vi "FABR-Init Hardware.vi"(0 "Stimulus":T1={"Ear"=enum."Left", "Start (kHz)"=0.0, "Stop (kHz)"=16.0, "Step (oct)"=5.0, "Start (dB)"=20, "Stop (dB)"=80, "Step (dB)"=5, "Rep rate (/sec)"=30.0, "Alternate Polarity"=FALSE, "Skip (oct)"=0.0} {"Start (kHz)" step=5.0; "Start (dB)" step=5}, 9 "Hidden":T3={"AI Samp Rate Hz"=25000.0, "AO Samp Rate Hz"=100000.0, "Duration (ms)"=5.0, "Ramp (ms)"=0.5, "Frame size (s)"=0.0}, 11 "error in (no error)":errorcluster) -> (4 "Stimulus thru":T1={"Ear"=enum."Left", "Start (kHz)"=0.0, "Stop (kHz)"=16.0, "Step (oct)"=5.0, "Start (dB)"=20, "Stop (dB)"=80, "Step (dB)"=5, "Rep rate (/sec)"=30.0, "Alternate Polarity"=FALSE, "Skip (oct)"=0.0} {"Start (kHz)" step=5.0; "Start (dB)" step=5}, 6 "Runtime":T2, 8 "Coerced rep rate":dbl, 15 "error out":errorcluster)   [LabVIEW 2020]
uses:
  Typedefs/FABR-Hidden Params.ctl
  Typedefs/FABR-Stimulus.ctl
  Typedefs/FABR-Runtime Data.ctl
  epl-vi-lib/Connection VIs/Type Defs/Input sources.ctl
  epl-vi-lib/Connection VIs/Type Defs/Output sources.ctl
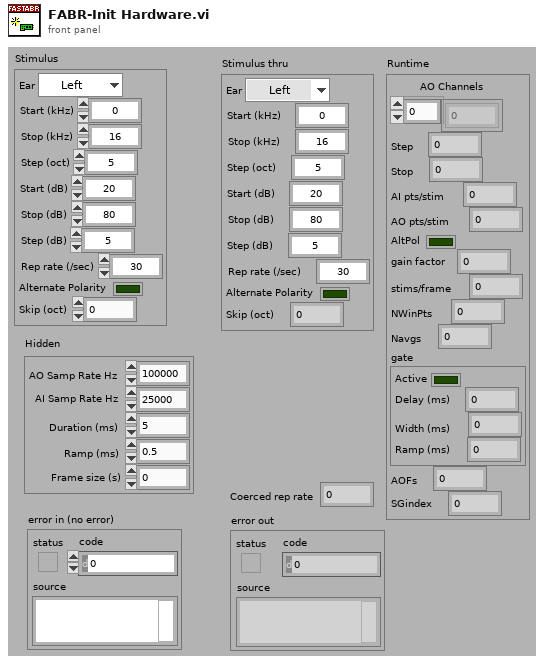
[diagram p1: front panel]
types:
  T1 = typedef "FABR-Stimulus.ctl" = cluster{"Ear":enum16{"Right", "Left"}, "Start (kHz)":dbl, "Stop (kHz)":dbl, "Step (oct)":dbl, "Start (dB)":i32, "Stop (dB)":i32, "Step (dB)":i32, "Rep rate (/sec)":dbl, "Alternate Polarity":bool, "Skip (oct)":dbl}
  T2 = typedef "FABR-Runtime Data.ctl" = cluster{"AO Channels":i32[], "Step":dbl, "Stop":i32, "AI pts/stim":i32, "AO pts/stim":i32, "AltPol":bool, "gain factor":dbl, "stims/frame":i32, "NWinPts":i32, "Navgs":i32, "gate":cluster{"Active":bool, "Delay (ms)":dbl, "Width (ms)":dbl, "Ramp (ms)":dbl}, "AOFs":dbl, "SGindex":i32}
  T3 = typedef "FABR-Hidden Params.ctl" = cluster{"AI Samp Rate Hz":dbl, "AO Samp Rate Hz":dbl, "Duration (ms)":dbl, "Ramp (ms)":dbl, "Frame size (s)":dbl}
  T4 = typedef "Input sources.ctl" = u16
  T5 = typedef "Output sources.ctl" = u16
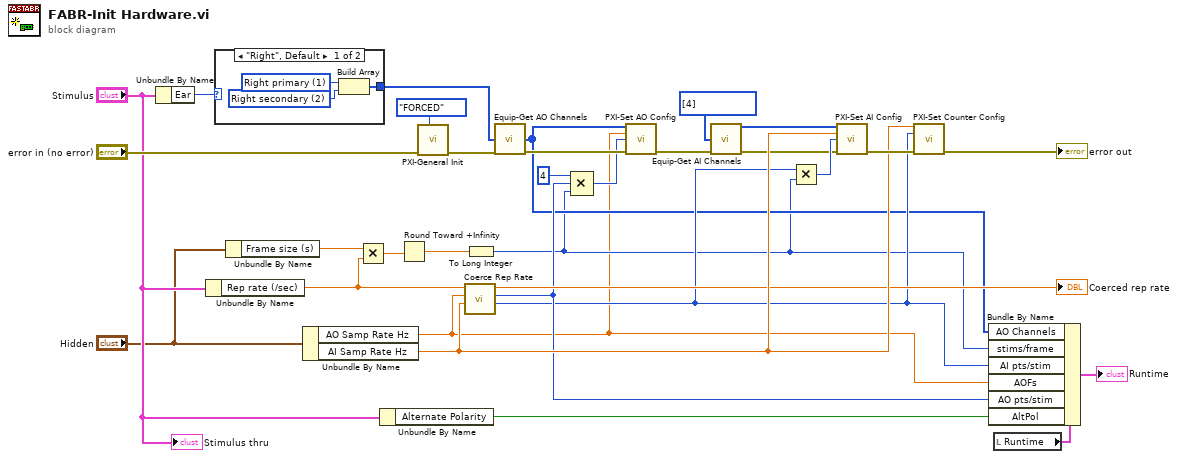
[diagram p0: block diagram]
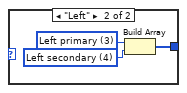
[diagram p2: hidden frame]
diagram:
  w9 = T4[] [4] items=["--unused--", "Probe Mic Right", "Probe Mic Left", "Cal Mic", "ABR", "CAP Right", "CAP Left", "Startle piezo", "Temperature", "Heart rate"]
  n1 = Unbundle By Name("Stimulus") -> ("Ear"=w22:enum16{"Right", "Left"})
  n2 = Unbundle By Name("Stimulus") -> ("Rep rate (/sec)"=w15:dbl)
  n3 = case shown="\"Right\", Default" w22 {
    tunnel: [w32 w35] -> w12
    frame "Right", Default {
      w33 = T5 2 items=["--unused--", "Right primary", "Right secondary", "Left primary", "Left secondary", "Shocks", "Startle", "Background"] ("Ring")
      w34 = T5 1 items=["--unused--", "Right primary", "Right secondary", "Left primary", "Left secondary", "Shocks", "Startle", "Background"] ("Ring")
      n4 = Build Array(w34, w33) -> (w32:T5[])
    }
    frame "Left" {
      w36 = T5 4 items=["--unused--", "Right primary", "Right secondary", "Left primary", "Left secondary", "Shocks", "Startle", "Background", "Shaker"] ("Ring")
      w37 = T5 3 items=["--unused--", "Right primary", "Right secondary", "Left primary", "Left secondary", "Shocks", "Startle", "Background"] ("Ring")
      n5 = Build Array(w37, w36) -> (w35:T5[])
    }
  }
  n6 = Unbundle By Name("Hidden") -> ("Frame size (s)"=w10:dbl)
  n7 = Unbundle By Name("Hidden") -> ("AO Samp Rate Hz"=w1:dbl, "AI Samp Rate Hz"=w25:dbl)
  n8 = Multiply(x=w10, y=w15) -> (x*y=w3:dbl)
  n9 = Unbundle By Name("Stimulus") -> ("Alternate Polarity"=w16:bool)
  n10 = Round Toward +Infinity(x=w3) -> (ceil(x): smallest int >= x=w2:dbl)
  n11 = call "PXI-General Init.vi"("Double Buffer Mode"=enum32{"OFF", "ENABLED", "FORCED"}."FORCED", "error in (no error)"="error in (no error)") -> ("error out"=w8:errorcluster)  [unwired: 9 in]
  n12 = call "Coerce Rep Rate.vi"("AI sampling rate (Hz)"=w25, "AO sampling rate (Hz)"=w1, "Rep rate (Hz)"=w15) -> ("AI npts"=w14:i32, "AO npts"=w21:i32, "Coerced rep rate (Hz)"=→"Coerced rep rate":dbl)  [unwired: 5 in, 1 out]
  n13 = To Long Integer(number=w2) -> (32bit integer=w4:i32)
  n14 = call "Equip-Get AO Channels.vi"("Outputs"=w12, "error in (no error)"=w8) -> ("AO Channels"=w5:i32[], "error out"=w29:errorcluster)  [unwired: 12 in]
  n15 = Compound Arithmetic op=MULTIPLY(4 ("x"), w21, w4) -> (w28:i32)
  n16 = call "PXI-Set AO Config.vi"("AO Channels"=w5, "Sampling Rate (Hz)"=w1, "Buffer Size"=w28, "error in (no error)"=w29) -> ("error out"=w7:errorcluster)  [unwired: 11 in]
  n17 = call "Equip-Get AI Channels.vi"("Inputs"=w9, "error in (no error)"=w7) -> ("AI Channels"=w20:i32[], "error out"=w6:errorcluster)  [unwired: 12 in]
  n18 = Multiply(x=w14, y=w4) -> (x*y=w13:i32)
  n19 = call "PXI-Set AI Config.vi"("AI Channels"=w20, "Sampling Rate (Hz)"=w25, "Buffer Size"=w13, "error in (no error)"=w6) -> ("error out"=w27:errorcluster)  [unwired: 11 in]
  n20 = call "PXI-Set Counter Config.vi"("AI Sampling Rate (Hz)"=w25, "Num AI Pts"=w14, "error in (no error)"=w27) -> ("error out"=→"error out":errorcluster)  [unwired: 12 in]
  n21 = local read "Runtime"() -> (w19:T2)
  n22 = Bundle By Name(cluster=w19, "AO Channels"=w5, "stims/frame"=w4, "AI pts/stim"=w14, "AOFs"=w1, "AO pts/stim"=w21, "AltPol"=w16) -> (→"Runtime":T2)
  "Stimulus thru" <- "Stimulus"
